vi "RTP_RTSP - Get Parameter (string).vi"(2 "Name":string, 7 "Data":string) -> (8 "Parameter":string)   [LabVIEW 2014]
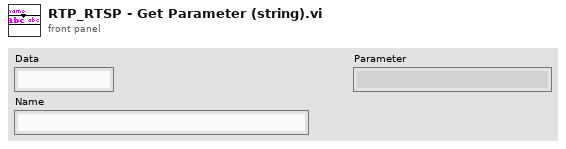
[diagram p1: front panel]
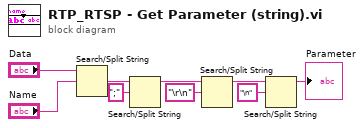
[diagram p0: block diagram]
diagram:
  n1 = Search/Split String(string="Data", search string/char (-)="Name") -> (match + rest of string=w8:string)  [unwired: 1 in, 2 out]
  n2 = Search/Split String(string=w8, search string/char (-)=";") -> (substring before match=w7:string)  [unwired: 1 in, 2 out]
  n3 = Search/Split String(string=w7, search string/char (-)="\r\n") -> (substring before match=w5:string)  [unwired: 1 in, 2 out]
  n4 = Search/Split String(string=w5, search string/char (-)="\n") -> (substring before match=→"Parameter":string)  [unwired: 1 in, 2 out]
